vi "Call Power On-Off.vi"(3 "error in":errorcluster, 4 "Warmup if ON":bool, 5 "VISA Ref In":refnum<visa-resource-name>, 6 "On/Off":bool=TRUE) -> (0 "error out":errorcluster, 1 "VISA Ref Out":refnum<visa-resource-name>)   [LabVIEW 2012]
doc: "The Basic Serial Read and Write example performs a Serial Port Read, a Serial Port Write, or a combination of these actions. The user selects the actions (read or write) on the front panel. If both are selected, the VI will write the data first, read data, and then close the VISA session that is opened to the port. This VI will wait until the specified number of bytes is received at the port or until a termination character is read.\n\nINSTRUCTIONS:\n1) Select the serial resource and configuration parameters (baud rate, data bits, parity, stop bits, flow control).\n2) Select the operations to be performed. \n3) Connect the serial port to your device. If no device is available, perform a loopback test by doing one of the following. Short pins 2 and 3 on a RS-232 cable or short pin 4 to pin 8 and pin 5 to pin 9 on a RS-485/422 cable. \n4) Run the VI to see the data read. (The \"read string\" will match the \"string to write\" if a loopback test was performed.)\n\nNote: The parameters set for the serial port must match the parameters of the connected instrument or device. In this example, the bytes to read parameter specifies the number of bytes that the serial port reads. If there were more bytes at the port than the number specified in bytes to read, those bytes would not be read. Also, if you specify to read more bytes than the number of bytes actually read, you might receive a timeout error message.\n\nOn the block diagram, the Configure Serial Port VI sets the configuration parameters. The front panel displays the controls used to configure the basic parameters, such as baud rate, data bits, and parity. Constants configure the other parameters the user probably does not need set. After the VISA Configure Serial Port VI opens the VISA session and configures the port, the VI passes the VISA resource name to other VIs that perform operations on that VISA resource. The VISA Write function sends a command to the serial device and the VISA Read function returns data based on the command. The VISA Close function then closes the reference to the serial device. It is important to close the reference; otherwise communication through with that port through protocols other than VISA might not be possible."
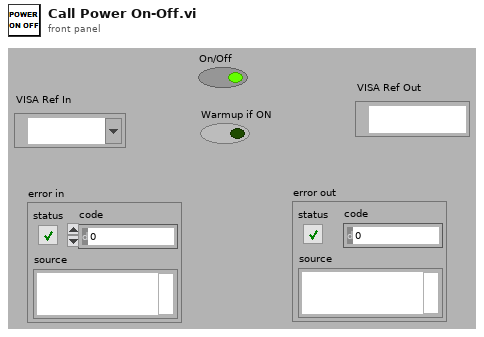
[diagram p1: front panel]
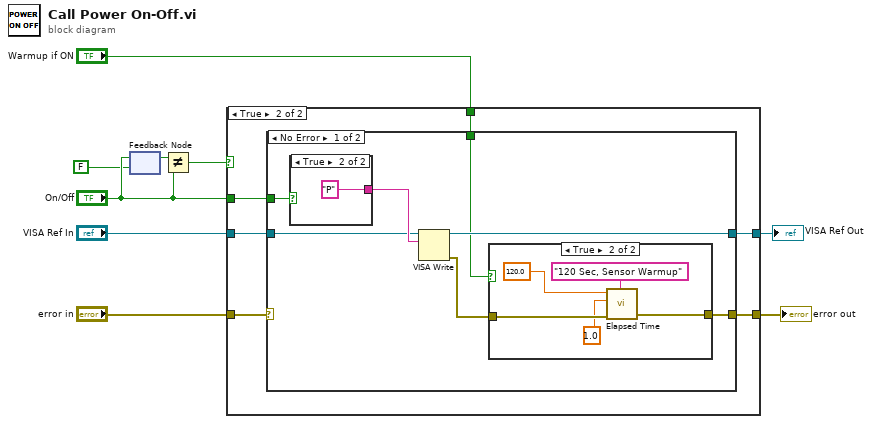
[diagram p0: block diagram]
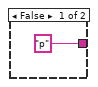
[diagram p4: hidden frame]
diagram:
  n1 = feedback-in #1("On/Off") -> ()
  n2 = feedback #1(FALSE ("On/Off")) -> (w4:bool)
  n3 = Not Equal?(x=w4, y="On/Off") -> (x != y?=w2:bool)
  n4 = case shown="True" w2 {
    tunnel: [w11 w17] -> w9
    tunnel: "VISA Ref In" -> [w11 w16]
    tunnel: [w10 w15] -> w7
    tunnel: "error in" -> [w10 w14]
    tunnel: "On/Off" -> [_ w13]
    tunnel: "Warmup if ON" -> [_ w12]
    frame False {
      # "If power is already on or off, do nothing."
    }
    frame True {
      n5 = case shown="No Error" w14 {
        selector: w14 -> [_ w33]
        tunnel: [w21 w34] -> w17
        tunnel: w16 -> [w23 w34]
        tunnel: [w20 w33] -> w15
        tunnel: w13 -> [w19 _]
        tunnel: w12 -> [w18 _]
        frame No Error {
          n6 = case shown="True" w19 {
            tunnel: ["p" "P"] -> w24
            frame False {
            }
            frame True {
            }
          }
          n7 = VISA Write(VISA resource name=w23, write buffer=w24) -> (VISA resource name out=w21:refnum<visa-resource-name>, error out=w22:errorcluster)  [unwired: 1 in, 1 out]
          n8 = case shown="True" w18 {
            tunnel: w22 -> [w25 w30]
            tunnel: [w25 w29] -> w20
            frame False {
            }
            frame True {
              n9 = call "Elapsed Time.vi"("error in (no error)"=w30, "Title"="120 Sec, Sensor Warmup", "Increment"=1.0, "Time Target (s)"=120.0) -> ("error out"=w29:errorcluster)  [unwired: 2 in]
            }
          }
        }
        frame Error {
        }
      }
    }
  }
  "error out" <- w7
  "VISA Ref Out" <- w9
